vi "UsrProfiles-Save changes-STRING.vi"(8 "error in (no error)":errorcluster, 10 "Keys of changed parameters-STRING":T2, 11 "User profile ini file ref":T1) -> (0 "error out":errorcluster, 3 "User profile ini file ref":T1)   [LabVIEW 2013]
uses:
  Typedefs/Changes info cluster-STRING.ctl
  Configuration code/Typedefs/Ini file interface (String).ctl
  <vilib>/Utility/config.llb/Config Data RefNum.ctl
  <vilib>/Utility/config.llb/NI_LVConfig.lvlib
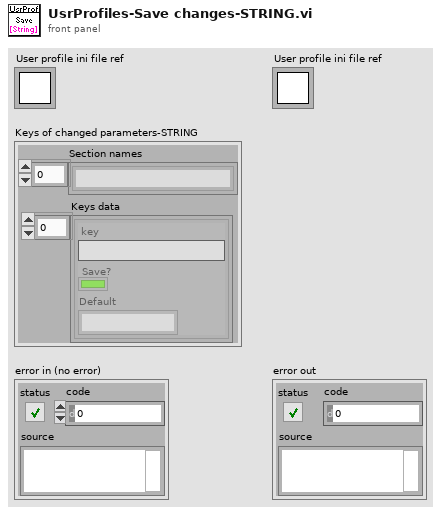
[diagram p1: front panel]
types:
  T1 = typedef "NI_LVConfig.lvlib/Config Data RefNum.ctl" = refnum<k1>
  T2 = typedef "Changes info cluster-STRING.ctl" = cluster{"Section names":string[], "Keys data":T3}
  T3 = typedef "Ini file interface (String).ctl" = cluster{"key":string, "Save?":bool, "Default":string}[]
  T4 = cluster{"key":string, "Save?":bool, "Default":string}[]
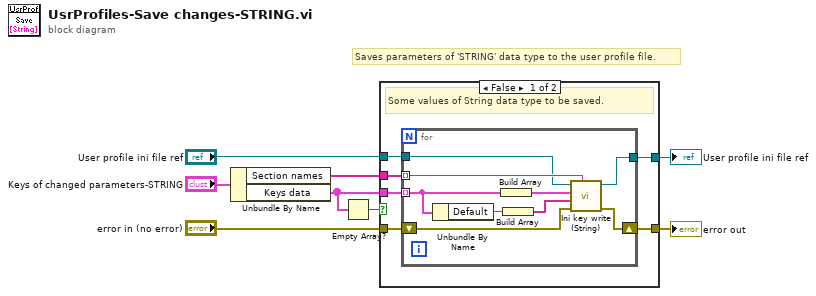
[diagram p0: block diagram]
diagram:
  # "Saves parameters of 'STRING' data type to the user profile file."
  n1 = Unbundle By Name("Keys of changed parameters-STRING") -> ("Section names"=w4:string[], "Keys data"=w2:T3)
  n2 = Empty Array?(array=w2) -> (empty?=w1:bool)
  n3 = case shown="False" w1 {
    tunnel: "error in (no error)" -> [w14 w24]
    tunnel: [w13 w24] -> w6
    tunnel: [w12 w25] -> w5
    tunnel: w2 -> [w11 _]
    tunnel: w4 -> [w10 _]
    tunnel: "User profile ini file ref" -> [w9 w25]
    frame False {
      # "Some values of String data type to be saved."
      n4 = for {
        tunnel: w11 -> [w17] mode=indexing
        tunnel: w10 -> [w22] mode=indexing
        shift-right: [w20] -> w13
        shift-left: w14 -> [w21]
        tunnel: w9 -> [w19]
        tunnel: [w18] -> w12
        n5 = Unbundle By Name(w17) -> ("Default"=w16:string)
        n6 = Build Array(w17) -> (w23:T4)
        n7 = Build Array(w16) -> (w15:string[])
        n8 = call "Ini key write (String).vi"("Section"=w22, "error in (no error)"=w21, "Values (String)"=w15, "Ini file interface"=w23, "Ini file refnum in"=w19) -> ("error out"=w20:errorcluster, "Ini file refnum out"=w18:T1)  [unwired: 5 in]
      }
    }
    frame True {
      # "No values of String data type to be saved."
    }
  }
  "error out" <- w6
  "User profile ini file ref" <- w5
